vi "CRYCurve Resolution.vi"(6 "smoothing":bool=TRUE, 8 "1/nOct_Hz":u32 caption="1/n Octave" step=1, 9 "Frequencies":u16(slide) caption="Freq Mode", 10 "New Resolution":u16(ring) items=["1/1 Octave", "1/3 Octave", "1/6 Octave", "1/12 Octave", "1/24 Octave", "User Defined log", "User Defined lin"], 11 "Curve in":T1={"Name"="", "Curve"=[], "X data"=1, "Y data"=1, "Z data"=1, "X axis"=0, "Y axis"=1, "Z axis"=1, "X unit"="Hz", "Y unit"="", "Z unit"="deg.", "X dB ref"=1.0, "Y dB ref"=1.0, "Z dB ref"=1.0, "single val"=FALSE, "protected"=FALSE, "display X"=TRUE, "display Y"=TRUE, "display Z"=TRUE, "Test Info"="", "Step No."=0, "Plot Settings"={"Color"=0, "Interpolation"=0, "Point Style"=0, "Line Style"=0, "Point Color"=0, "Line Width"=0, "Bar Plot Style"=0, "Fill To"=0}, "AutoProtect"=FALSE} {"Z data" items=["dB", "Lin"]; "X data" items=["dB", "Lin"]; "Y data" items=["dB", "Lin"]; "Z dB ref" format="%.1f"; "Z axis" items=["Log", "Lin"]; "X dB ref" format="%.1f"; "X axis" items=["Log", "Lin"]; "Y axis" items=["Log", "Lin"]; "Y dB ref" format="%.1f"; "Curve"."z" format="%.2f"; "Curve"."y" format="%.2f"; "Curve"."x" format="%.2f"}) -> (3 "Curve out":T1={"Name"="", "Curve"=[], "X data"=1, "Y data"=1, "Z data"=1, "X axis"=0, "Y axis"=1, "Z axis"=1, "X unit"="Hz", "Y unit"="", "Z unit"="deg.", "X dB ref"=1.0, "Y dB ref"=1.0, "Z dB ref"=1.0, "single val"=FALSE, "protected"=FALSE, "display X"=TRUE, "display Y"=TRUE, "display Z"=TRUE, "Test Info"="", "Step No."=0, "Plot Settings"={"Color"=0, "Interpolation"=0, "Point Style"=0, "Line Style"=0, "Point Color"=0, "Line Width"=0, "Bar Plot Style"=0, "Fill To"=0}, "AutoProtect"=FALSE} {"Z data" items=["dB", "Lin"]; "X data" items=["dB", "Lin"]; "Y data" items=["dB", "Lin"]; "Z dB ref" format="%.1f"; "Z axis" items=["Log", "Lin"]; "X dB ref" format="%.1f"; "X axis" items=["Log", "Lin"]; "Y axis" items=["Log", "Lin"]; "Y dB ref" format="%.1f"; "Curve"."z" format="%.2f"; "Curve"."y" format="%.2f"; "Curve"."x" format="%.2f"})   [LabVIEW 2013]
uses:
  Typedef Control/CRYData Cluster.ctl
  Stimulus/SubVI/CRYStimulus Global.vi
panel:
  in  "smoothing 2":bool=TRUE
  in  "RTA R20(1/12) series":dbl[](array[numeric])=[1.0, 1.1, 1.1, 1.2, 1.3, 1.4, 1.4, 1.5, 1.6, 1.7, 1.8, 1.9, 2.0, 2.2, 2.3, 2.4, 2.6, 2.7, 2.9, 3.0, 3.2, 3.4, 3.6, 3.8, 4.1, 4.3, 4.6, 4.8, 5.1, 5.4, 5.8, 6.1, 6.5, 6.8, 7.2, 7.7, 8.1, 8.6, 9.1, 9.7, 10.2, 10.9, 11.5, 12.2, 12.9, 13.7, 14.5, 15.4, 16.3, 17.3, 18.3, 19.4, 20.5, 21.8, 23.0, 24.4, 25.9, 27.4, 29.0, 30.7, 32.5, 34.5, 36.5, 38.7, 41.0, 43.4, 46.0, 48.7, 51.6, 54.6, 57.9, 61.3, 64.9, 68.8, 72.9, 77.2, 81.8, 86.6, 91.7, 97.2, 103.0, 109.0, 115.0, 122.0, 130.0, 137.0, 145.0, 154.0, 163.0, 173.0, 183.0, 194.0, 205.0, 218.0, 230.0, 244.0, 259.0, 274.0, 290.0, 307.0, 325.0, 345.0, 365.0, 387.0, 410.0, 434.0, 460.0, 487.0, 516.0, 546.0, 579.0, 613.0, 649.0, 688.0, 729.0, 772.0, 818.0, 866.0, 917.0, 972.0, 1030.0, 1090.0, 1150.0, 1220.0, 1300.0, 1370.0, 1450.0, 1540.0, 1630.0, 1730.0, 1830.0, 1940.0, 2050.0, 2180.0, 2300.0, 2440.0, 2590.0, 2740.0, 2900.0, 3070.0, 3250.0, 3450.0, 3650.0, 3870.0, 4100.0, 4340.0, 4600.0, 4870.0, 5160.0, 5460.0, 5790.0, 6130.0, 6490.0, 6880.0, 7290.0, 7720.0, 8180.0, 8660.0, 9170.0, 9720.0, 10300.0, 10900.0, 11500.0, 12200.0, 13000.0, 13700.0, 14500.0, 15400.0, 16300.0, 17300.0, 18300.0, 19400.0, 20500.0] format="%.2f"
  in  "RTA R20(1/6) series":dbl[](array[numeric])=[1.05, 1.17, 1.32, 1.48, 1.66, 1.86, 2.09, 2.35, 2.64, 2.96, 3.32, 3.73, 4.19, 4.7, 5.28, 5.92, 6.65, 7.46, 8.37, 9.4, 10.55, 11.84, 13.29, 14.92, 16.8, 18.8, 21.1, 23.7, 26.6, 29.9, 33.5, 37.6, 42.2, 47.3, 53.1, 59.6, 66.8, 75.0, 84.1, 94.4, 106.0, 119.0, 133.0, 150.0, 168.0, 188.0, 211.0, 237.0, 266.0, 299.0, 335.0, 376.0, 422.0, 473.0, 531.0, 596.0, 668.0, 750.0, 841.0, 944.0, 1060.0, 1190.0, 1330.0, 1500.0, 1680.0, 1880.0, 2110.0, 2370.0, 2660.0, 2990.0, 3350.0, 3760.0, 4220.0, 4730.0, 5310.0, 5960.0, 6680.0, 7500.0, 8410.0, 9440.0, 10600.0, 11900.0, 13300.0, 15000.0, 16801.0, 18800.0, 21100.0] format="%.2f"
  in  "RTA R80(1/24) series":dbl[](array[numeric])=[1.01, 1.0299999713897705, 1.07, 1.1, 1.13, 1.17, 1.2, 1.24, 1.27, 1.31, 1.35, 1.39, 1.43, 1.47, 1.51, 1.56, 1.600000023841858, 1.649999976158142, 1.7000000476837158, 1.75, 1.7999999523162842, 1.850000023841858, 1.899999976158142, 1.96, 2.02, 2.07, 2.13, 2.2, 2.26, 2.33, 2.4, 2.46, 2.54, 2.61, 2.69, 2.77, 2.85, 2.9000000953674316, 3.0, 3.1, 3.2, 3.3, 3.4, 3.5, 3.6, 3.7, 3.8, 3.9, 4.0, 4.1, 4.3, 4.4, 4.5, 4.6, 4.8, 4.9, 5.0, 5.2, 5.4, 5.5, 5.7, 5.800000190734863, 6.0, 6.2, 6.4, 6.6, 6.8, 7.0, 7.2, 7.4, 7.6, 7.8, 8.0, 8.3, 8.5, 8.7, 9.0, 9.3, 9.5, 9.8, 10.1, 10.4, 10.7, 11.1, 11.4, 11.7, 12.1, 12.4, 12.8, 13.1, 13.5, 13.9, 14.3, 14.7, 15.2, 15.6, 16.1, 16.5, 17.0, 17.5, 18.0, 18.6, 19.1, 19.7, 20.2, 20.8, 21.4, 22.1, 22.7, 23.4, 24.1, 24.8, 25.5, 26.2, 27.0, 27.8, 28.6, 29.4, 30.3, 31.2, 32.1, 33.0, 34.0, 35.0, 36.0, 37.0, 38.1, 39.2, 40.4, 41.6, 42.8, 44.0, 45.3, 46.6, 48.0, 49.4, 50.8, 52.3, 53.9, 55.4, 57.0, 58.7, 60.4, 62.2, 64.0, 65.9, 67.8, 69.8, 71.8, 73.9, 76.1, 78.3, 80.6, 82.9, 85.4, 87.9, 90.4, 93.1, 95.8, 98.6, 101.0, 104.0, 107.0, 111.0, 114.0, 117.0, 121.0, 124.0, 128.0, 131.0, 135.0, 139.0, 143.0, 147.0, 152.0, 156.0, 161.0, 165.0, 170.0, 175.0, 180.0, 186.0, 191.0, 197.0, 202.0, 208.0, 214.0, 221.0, 227.0, 234.0, 241.0, 248.0, 255.0, 262.0, 270.0, 278.0, 286.0, 294.0, 303.0, 312.0, 321.0, 330.0, 340.0, 350.0, 360.0, 370.0, 381.0, 392.0, 404.0, 416.0, 428.0, 440.0, 453.0, 466.0, 480.0, 494.0, 508.0, 523.0, 539.0, 554.0, 570.0, 587.0, 604.0, 622.0, 640.0, 659.0, 678.0, 698.0, 718.0, 739.0, 761.0, 783.0, 806.0, 829.0, 854.0, 879.0, 904.0, 931.0, 958.0, 986.0, 1010.0, 1040.0, 1070.0, 1110.0, 1140.0, 1170.0, 1210.0, 1240.0, 1280.0, 1310.0, 1350.0, 1390.0, 1430.0, 1470.0, 1520.0, 1560.0, 1610.0, 1650.0, 1700.0, 1750.0, 1800.0, 1860.0, 1910.0, 1970.0, 2020.0, 2080.0, 2140.0, 2210.0, 2270.0, 2340.0, 2410.0, 2480.0, 2550.0, 2620.0, 2700.0, 2780.0, 2860.0, 2940.0, 3030.0, 3120.0, 3210.0, 3300.0, 3400.0, 3500.0, 3600.0, 3700.0, 3810.0, 3920.0, 4040.0, 4160.0, 4280.0, 4400.0, 4530.0, 4660.0, 4800.0, 4940.0, 5080.0, 5230.0, 5390.0, 5540.0, 5700.0, 5870.0, 6040.0, 6220.0, 6400.0, 6590.0, 6780.0, 6980.0, 7180.0, 7390.0, 7610.0, 7830.0, 8060.0, 8290.0, 8540.0, 8790.0, 9040.0, 9310.0, 9580.0, 9860.0, 10100.0, 10400.0, 10700.0, 11100.0, 11400.0, 11700.0, 12100.0, 12400.0, 12800.0, 13100.0, 13500.0, 13900.0, 14300.0, 14700.0, 15200.0, 15600.0, 16100.0, 16500.0, 17000.0, 17500.0, 18000.0, 18600.0, 19100.0, 19700.0, 20200.0, 20800.0, 21400.0, 22100.0, 22700.0, 23400.0, 24100.0, 24800.0, 25500.0, 26200.0, 27000.0, 27800.0, 28600.0, 29400.0, 30300.0, 31200.0, 32100.0, 33000.0, 34000.0, 35000.0, 36000.0, 37000.0, 38100.0, 39200.0, 40400.0, 41600.0, 42800.0, 44000.0, 45300.0, 46600.0, 48000.0, 49400.0, 50800.0, 52300.0, 53900.0, 55400.0, 57000.0, 58700.0, 60400.0, 62200.0, 64000.0, 65900.0, 67800.0, 69800.0, 71800.0, 73900.0, 76100.0, 78300.0, 80600.0, 82900.0, 85400.0, 87900.0, 90400.0, 93100.0, 95800.0, 98600.0] format="%.2f"
  out "Freq":dbl[](array[numeric])
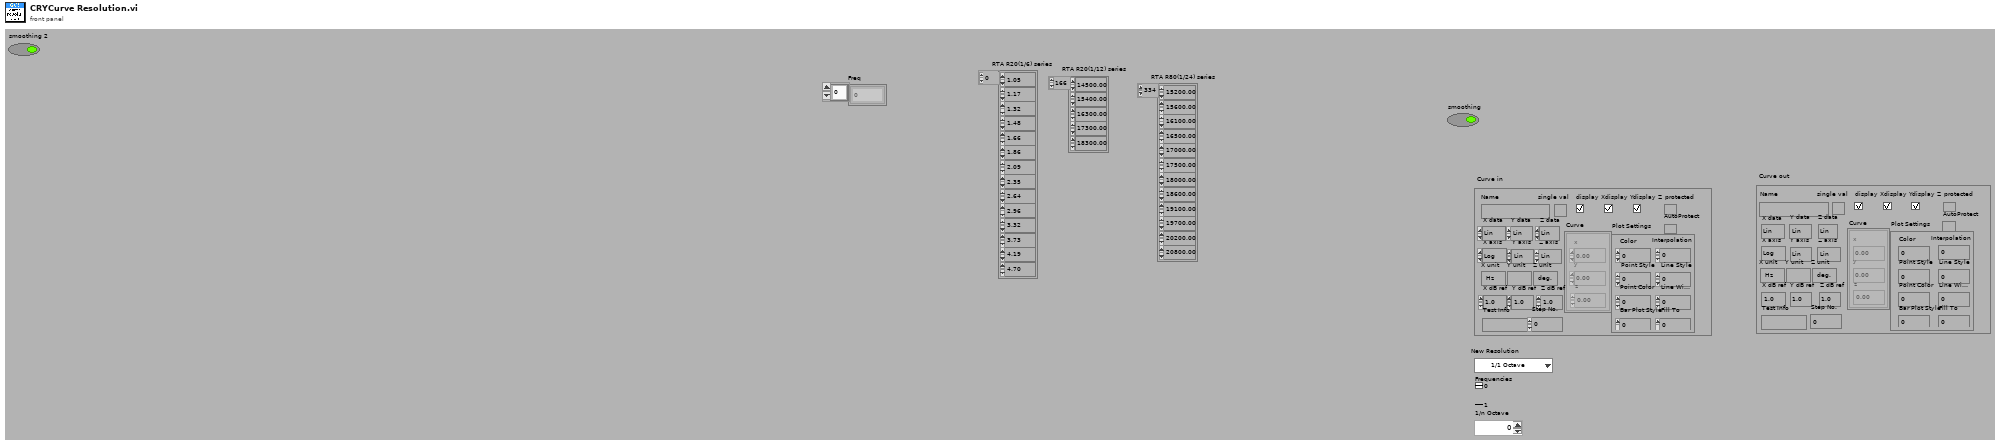
[diagram p1: front panel]
types:
  T1 = typedef "CRYData Cluster.ctl" = cluster{"Name":string, "Curve":cluster{"x":dbl, "y":dbl, "z":dbl}[], "X data":u16, "Y data":u16, "Z data":u16, "X axis":u16, "Y axis":u16, "Z axis":u16, "X unit":string, "Y unit":string, "Z unit":string, "X dB ref":dbl, "Y dB ref":dbl, "Z dB ref":dbl, "single val":bool, "protected":bool, "display X":bool, "display Y":bool, "display Z":bool, "Test Info":string, "Step No.":i32, "Plot Settings":cluster{"Color":u32, "Interpolation":u8, "Point Style":u8, "Line Style":u8, "Point Color":u32, "Line Width":u8, "Bar Plot Style":u8, "Fill To":i16}, "AutoProtect":bool}
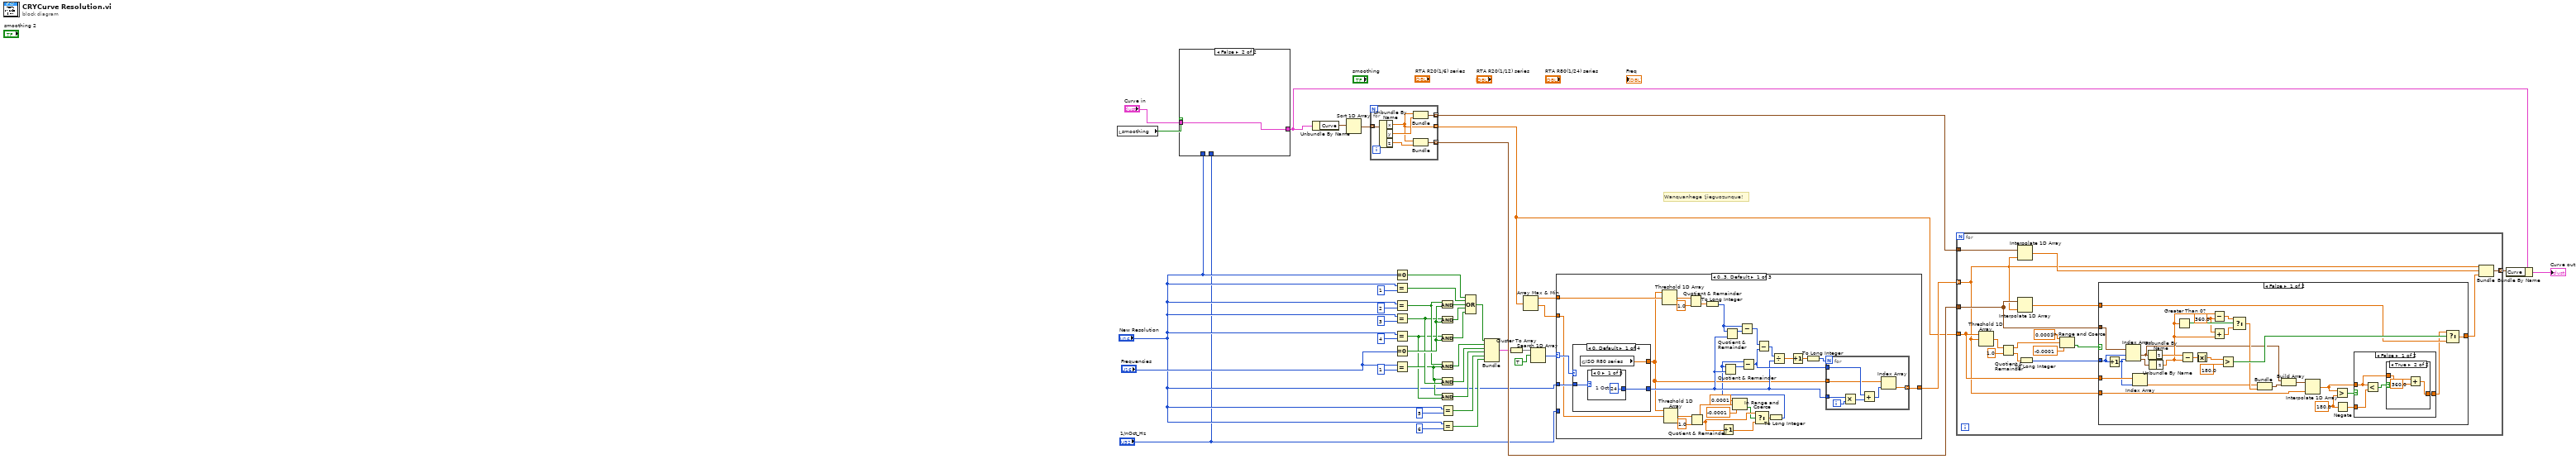
[diagram p0: block diagram]
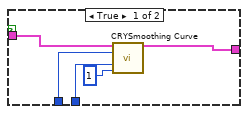
[diagram p2: hidden frame]
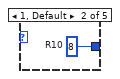
[diagram p3: hidden frame]
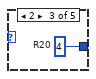
[diagram p4: hidden frame]
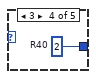
[diagram p5: hidden frame]
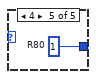
[diagram p6: hidden frame]
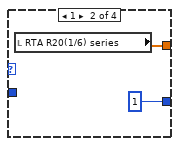
[diagram p7: hidden frame]
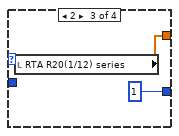
[diagram p8: hidden frame]
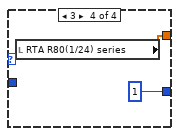
[diagram p9: hidden frame]
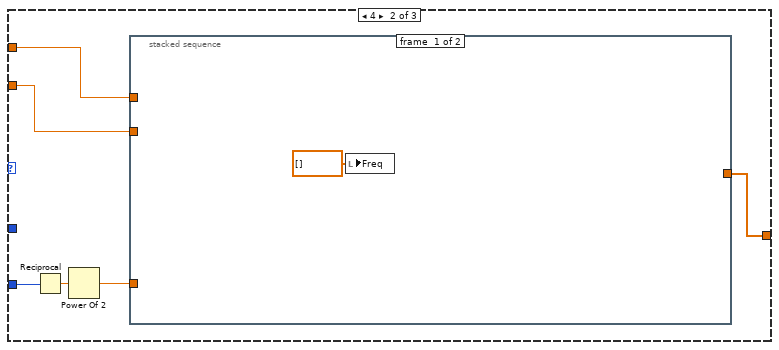
[diagram p10: hidden frame]
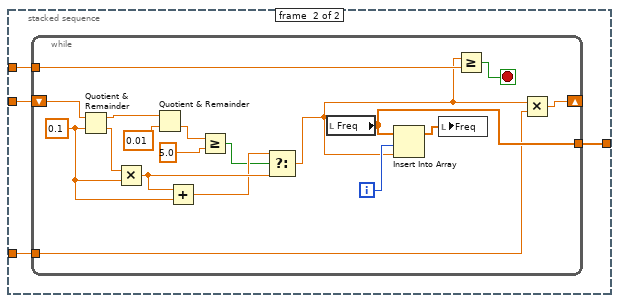
[diagram p11: hidden frame]
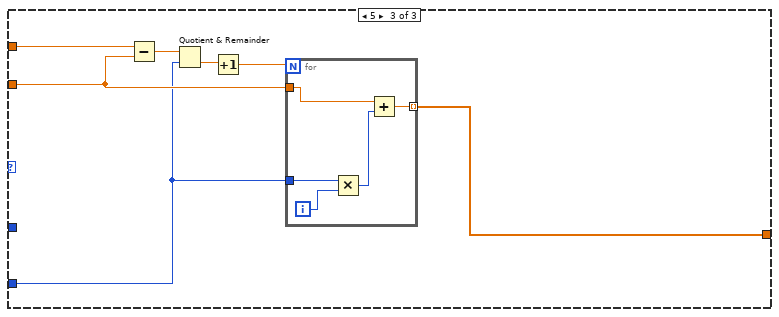
[diagram p12: hidden frame]
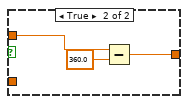
[diagram p14: hidden frame]
diagram:
  # "Wanquanhege !jieguozunque!"
  n1 = local read "smoothing"() -> (w6:bool)
  n2 = case shown="False" w6 {
    tunnel: "Curve in" -> [w47 w49]
    tunnel: "New Resolution" -> [w48 _]
    tunnel: [w44 w49] -> w3
    tunnel: "1/nOct_Hz" -> [w46 _]
    frame True {
      n3 = call "CRYSmoothing Curve.vi"("Data in"=w47, "Octav Mode"=w48, "Octave steps"=w46, "Weight Mode"=1) -> ("Resulting data out"=w44:T1)  [unwired: 2 in, 9 out]
    }
    frame False {
    }
  }
  n4 = Unbundle By Name(w3) -> ("Curve"=w10:cluster{"x":dbl, "y":dbl, "z":dbl}[])
  n5 = Sort 1D Array(array=w10) -> (sorted array=w41:cluster{"x":dbl, "y":dbl, "z":dbl}[])
  n6 = for {
    tunnel: w41 -> [w55] mode=indexing
    tunnel: [w52] -> w9 mode=indexing
    tunnel: [w53] -> w43 mode=indexing
    tunnel: [w50] -> w42 mode=indexing
    n7 = Unbundle By Name(w55) -> ("x"=w52:dbl, "y"=w54:dbl, "z"=w51:dbl)
    n8 = Bundle("x"=w52, "y"=w54) -> (w53:cluster{"x":dbl, "y":dbl})  [unwired: 1 out]
    n9 = Bundle("x"=w52, "z"=w51) -> (w50:cluster{"x":dbl, "z":dbl})  [unwired: 1 out]
  }
  n10 = Equal To 0?(x="New Resolution") -> (x = 0?=w35:bool)
  n11 = Equal?(x="New Resolution", y=u16 1) -> (x = y?=w34:bool)
  n12 = Equal?(x="New Resolution", y=u16 2) -> (x = y?=w29:bool)
  n13 = Equal?(x="New Resolution", y=u16 3) -> (x = y?=w28:bool)
  n14 = Equal?(x="New Resolution", y=u16 4) -> (x = y?=w26:bool)
  n15 = Equal To 0?(x="Frequencies") -> (x = 0?=w36:bool)
  n16 = Equal?(x="Frequencies", y=u16 1) -> (x = y?=w27:bool)
  n17 = And(x=w29, y=w36) -> (x .and. y?=w33:bool)
  n18 = And(x=w28, y=w36) -> (x .and. y?=w32:bool)
  n19 = And(x=w26, y=w36) -> (x .and. y?=w31:bool)
  n20 = And(x=w29, y=w27) -> (x .and. y?=w19:bool)
  n21 = And(x=w27, y=w28) -> (x .and. y?=w18:bool)
  n22 = And(x=w27, y=w26) -> (x .and. y?=w17:bool)
  n23 = Equal?(x="New Resolution", y=u16 5) -> (x = y?=w16:bool)
  n24 = Equal?(x="New Resolution", y=u16 6) -> (x = y?=w15:bool)
  n25 = Compound Arithmetic op=OR(w35, w34, w33, w32, w31) -> (w20:bool)
  n26 = Bundle(w20, w19, w18, w17, w16, w15) -> (w22:cluster{bool, bool, bool, bool, bool, bool})  [unwired: 1 out]
  n27 = Cluster To Array(cluster=w22) -> (array=w21:bool[])
  n28 = Array Max & Min(array=w9) -> (max value=w14:dbl, min value=w13:dbl)  [unwired: 2 out]
  n29 = Search 1D Array(1D array=w21, element=TRUE) -> (index of element=w12:i32)  [unwired: 1 out]
  n30 = case shown="0..3, Default" w12 {
    selector: w12 -> [w73 _ _]
    tunnel: "New Resolution" -> [w84 _ _]
    tunnel: w14 -> [w72 w111 w138]
    tunnel: w13 -> [w62 w110 w137]
    tunnel: [w74 w109 w135] -> w11
    tunnel: "1/nOct_Hz" -> [_ w107 w136]
    frame 0..3, Default {
      n31 = case shown="0, Default" w73 {
        tunnel: w84 -> [w87 _ _ _]
        tunnel: [w85 w94 w96 w97] -> w63
        tunnel: [w86 1 ("R80") 1 ("R80") 1 ("R80")] -> w75
        frame 0, Default {
          n32 = global read "CRYStimulus Global.vi" "ISO R80 series"() -> (w85:dbl[])
          n33 = case shown="0" w87 {
            tunnel: [w88 w89 w90 w91 w92] -> w86
            frame 0 {
              w88 = 24  # 1 Oct
            }
            frame 1, Default {
              w89 = 8  # R10
            }
            frame 2 {
              w90 = 4  # R20
            }
            frame 3 {
              w91 = 2  # R40
            }
            frame 4 {
              w92 = 1  # R80
            }
          }
        }
        frame 1 {
          n34 = local read "RTA R20(1/6) series"() -> (w94:dbl[])
        }
        frame 2 {
          n35 = local read "RTA R20(1/12) series"() -> (w96:dbl[])
        }
        frame 3 {
          n36 = local read "RTA R80(1/24) series"() -> (w97:dbl[])
        }
      }
      n37 = Threshold 1D Array(2:w72, 3:w63) -> (0:w71:dbl)  [unwired: 1 in]
      n38 = Threshold 1D Array(2:w62, 3:w63) -> (0:w64:dbl)  [unwired: 1 in]
      n39 = Quotient & Remainder(x=w71, y=1.0) -> (floor(x/y)=w56:dbl)  [unwired: 1 out]
      n40 = Quotient & Remainder(x=w64, y=1.0) -> (x-y*floor(x/y)=w58:dbl, floor(x/y)=w66:dbl)
      n41 = To Long Integer(number=w56) -> (32bit integer=w69:i32)
      n42 = Increment(x=w66) -> (x+1=w67:dbl)
      n43 = Quotient & Remainder(x=w69, y=w75) -> (x-y*floor(x/y)=w79:i32)  [unwired: 1 out]
      n44 = In Range and Coerce(upper limit=0.0001, x=w58, lower limit=-0.0001) -> (In Range?=w57:bool)  [unwired: 1 out]
      n45 = Subtract(x=w69, y=w79) -> (x-y=w80:i32)
      n46 = Select(t=w66, s=w57, f=w67) -> (s? t:f=w68:dbl)
      n47 = To Long Integer(number=w68) -> (32bit integer=w61:i32)
      n48 = Quotient & Remainder(x=w61, y=w75) -> (x-y*floor(x/y)=w78:i32)  [unwired: 1 out]
      n49 = Subtract(x=w61, y=w78) -> (x-y=w76:i32)
      n50 = Subtract(x=w80, y=w76) -> (x-y=w81:i32)
      n51 = Divide(x=w81, y=w75) -> (x/y=w82:dbl)
      n52 = Increment(x=w82) -> (x+1=w83:dbl)
      n53 = To Long Integer(number=w83) -> (32bit integer=w77:i32)
      n54 = for {
        N: w77 -> [_]
        tunnel: w76 -> [w103]
        tunnel: w75 -> [w102]
        tunnel: w63 -> [w100]
        tunnel: [w99] -> w74 mode=indexing
        i -> [w101]
        n55 = Multiply(x=w102, y=w101) -> (x*y=w104:i32)
        n56 = Add(x=w103, y=w104) -> (x+y=w105:i32)
        n57 = Index Array(array=w100, index=w105) -> (element=w99:dbl)
      }
    }
    frame 4 {
      n58 = Reciprocal(x=w107) -> (1/x=w108:dbl)
      n59 = Power Of 2(x=w108) -> (2^x=w106:dbl)
      n60 = stacked-sequence {
        tunnel: w110 -> [_ w116]
        tunnel: w106 -> [_ w115]
        tunnel: w111 -> [_ w114]
        tunnel: [_ w113] -> w109
        frame #0 {
          n61 = local write "Freq"(dbl[] [] ("Array")) -> ()
        }
        frame #1 {
          n62 = while {
            tunnel: w115 -> [w117]
            tunnel: w114 -> [w131]
            shift-right: [w134] -> _
            shift-left: w116 -> [w119]
            tunnel: [w129] -> w113
            i -> [w133]
            stop <- w132 stop-if-true
            w126 = 0.1 ("y")
            n63 = Quotient & Remainder(x=w119, y=w126) -> (x-y*floor(x/y)=w120:dbl, floor(x/y)=w122:dbl)
            n64 = Multiply(x=w122, y=w126) -> (x*y=w128:dbl)
            n65 = Quotient & Remainder(x=w120, y=0.01) -> (floor(x/y)=w123:dbl)  [unwired: 1 out]
            n66 = Add(x=w128, y=w126) -> (x+y=w127:dbl)
            n67 = Greater Or Equal?(x=w123, y=5.0) -> (x >= y?=w125:bool)
            n68 = Select(t=w127, s=w125, f=w128) -> (s? t:f=w118:dbl)
            n69 = local read "Freq"() -> (w129:dbl[])
            n70 = Insert Into Array(array=w129, index=w133, new element=w118) -> (w130:dbl[])
            n71 = local write "Freq"(w130) -> ()
            n72 = Greater Or Equal?(x=w118, y=w131) -> (x >= y?=w132:bool)
            n73 = Multiply(x=w118, y=w117) -> (x*y=w134:dbl)
          }
        }
      }
    }
    frame 5 {
      n74 = Subtract(x=w138, y=w137) -> (x-y=w139:dbl)
      n75 = Quotient & Remainder(x=w139, y=w136) -> (floor(x/y)=w140:dbl)  [unwired: 1 out]
      n76 = Increment(x=w140) -> (x+1=w141:dbl)
      n77 = for {
        N: w141 -> [_]
        tunnel: w137 -> [w146]
        tunnel: w136 -> [w144]
        tunnel: [w142] -> w135 mode=indexing
        i -> [w145]
        n78 = Multiply(x=w144, y=w145) -> (x*y=w143:u32)
        n79 = Add(x=w146, y=w143) -> (x+y=w142:dbl)
      }
    }
  }
  n80 = for {
    tunnel: w11 -> [w151] mode=indexing
    tunnel: w43 -> [w162]
    tunnel: w42 -> [w153]
    tunnel: [w160] -> w8 mode=indexing
    tunnel: w9 -> [w152]
    n81 = Threshold 1D Array(2:w151, 3:w152) -> (0:w159:dbl)  [unwired: 1 in]
    n82 = Quotient & Remainder(x=w159, y=1.0) -> (x-y*floor(x/y)=w148:dbl, floor(x/y)=w155:dbl)
    n83 = Interpolate 1D Array(1:w151, 2:w162) -> (0:w161:dbl)
    n84 = Interpolate 1D Array(1:w151, 2:w153) -> (0:w157:dbl)
    n85 = To Long Integer(number=w155) -> (32bit integer=w154:i32)
    n86 = In Range and Coerce(upper limit=0.0001, x=w148, lower limit=-0.0001) -> (In Range?=w147:bool)  [unwired: 1 out]
    n87 = case shown="False" w147 {
      tunnel: w157 -> [w168 w202]
      tunnel: [w184 w202] -> w156
      tunnel: w154 -> [w190 _]
      tunnel: w153 -> [w189 _]
      tunnel: w152 -> [w176 _]
      tunnel: w151 -> [w169 _]
      frame False {
        w166 = 180.0 ("y")
        w178 = 360.0 ("y")
        n88 = Increment(x=w190) -> (x+1=w175:i32)
        n89 = Index Array(array=w189, index #1=w190, index #2=w175) -> (element #1=w171:cluster{"x":dbl, "z":dbl}, element #2=w188:cluster{"x":dbl, "z":dbl})
        n90 = Index Array(array=w176, index=w175) -> (element=w173:dbl)
        n91 = Unbundle By Name(w171) -> ("z"=w187:dbl)
        n92 = Unbundle By Name(w188) -> ("z"=w177:dbl)
        n93 = Greater Than 0?(x=w177) -> (x > 0?=w182:bool)
        n94 = Subtract(x=w187, y=w177) -> (x-y=w186:dbl)
        n95 = Absolute Value(x=w186) -> (abs(x)=w185:dbl)
        n96 = Subtract(x=w177, y=w178) -> (x-y=w181:dbl)
        n97 = Add(x=w178, y=w177) -> (x+y=w179:dbl)
        n98 = Greater?(x=w185, y=180.0) -> (0:w183:bool)
        n99 = Select(t=w181, s=w182, f=w179) -> (s? t:f=w174:dbl)
        n100 = Bundle("x"=w173, w174) -> (w172:cluster{"x":dbl, dbl})  [unwired: 1 in]
        n101 = Build Array(w171, w172) -> (w170:cluster{"x":dbl, "z":dbl}[])
        n102 = Interpolate 1D Array(1:w169, 2:w170) -> (0:w164:dbl)
        n103 = Greater?(x=w164, y=w166) -> (0:w165:bool)
        n104 = Negate(x=w166) -> (-x=w167:dbl)
        n105 = case shown="False" w165 {
          tunnel: w164 -> [w192 w201]
          tunnel: [w191 w199] -> w163
          tunnel: w167 -> [w194 _]
          frame False {
            n106 = Less?(x=w192, y=w194) -> (x < y?=w193:bool)
            n107 = case shown="True" w193 {
              tunnel: w192 -> [w195 w198]
              tunnel: [w195 w196] -> w191
              frame False {
              }
              frame True {
                n108 = Add(x=w198, y=360.0) -> (x+y=w196:dbl)
              }
            }
          }
          frame True {
            n109 = Subtract(x=w201, y=360.0) -> (x-y=w199:dbl)
          }
        }
        n110 = Select(t=w163, s=w183, f=w168) -> (s? t:f=w184:dbl)
      }
      frame True {
      }
    }
    n111 = Bundle("Next Freq"=w151, w161, w156) -> (w160:cluster{"Next Freq":dbl, dbl, dbl})  [unwired: 1 out]
  }
  n112 = Bundle By Name(cluster=w3, "Curve"=w8) -> (→"Curve out":T1)
